vi "AlliGator ucno_objective function phasor calibration.vi"(3 "output control":T1, 4 "data":variant, 5 "X":dbl[](array[numeric])) -> (0 "error out":errorcluster, 1 "gradient":dbl[](array[numeric]), 2 "f(X)":dbl)   [LabVIEW 2021, in "AlliGator Phasor Calibration.lvlib"]
doc: "Minimization function used to search for the optimal calibration based on two references."
uses:
  Variant/Variant to Data/Variant to [DBL].vi
  AlliGator Phasor Calibration.lvlib
  Variant/Variant to Data/Variant to Data.lvlib
panel:
  # "see the AlliGator License on the block diagram (Ctrl+E or Window:Show Block Diagram)"
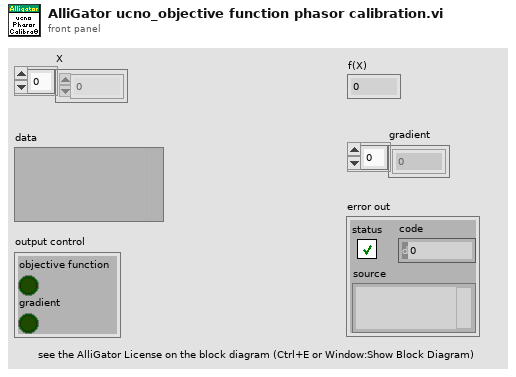
[diagram p1: front panel]
types:
  T1 = cluster{"objective function":bool, "gradient":bool}
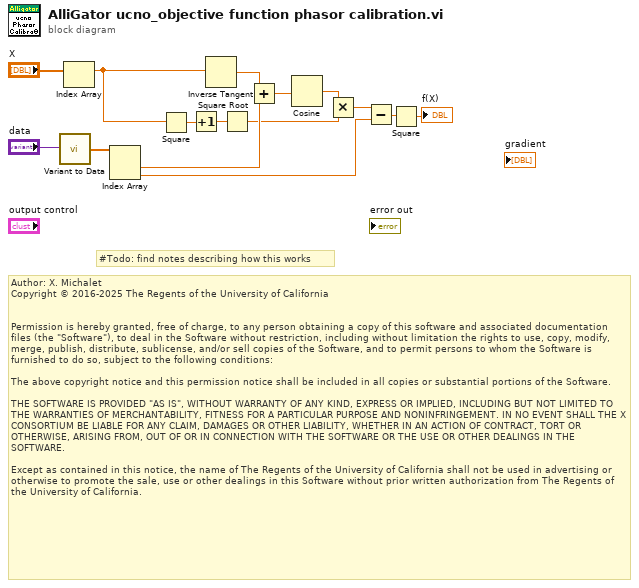
[diagram p0: block diagram]
diagram:
  # "Author: X. Michalet\nCopyright © 2016-2025 The Regents of the University of California\n \n\nPermission is hereby granted, free of charge, to any person obtaining a copy of this software and associated documentation files (the \"Software\"), to deal in the Software without restriction, including without limitation the rights to use, copy, modify, merge, publish, distribute, sublicense, and/or sell copies of the Software, and to permit persons to whom the Software is furnished to do so, subject to the following conditions:\n\nThe above copyright notice and this permission notice shall be included in all copies or substantial portions of the Software.\n\nTHE SOFTWARE IS PROVIDED \"AS IS\", WITHOUT WARRANTY OF ANY KIND, EXPRESS OR IMPLIED, INCLUDING BUT NOT LIMITED TO THE WARRANTIES OF MERCHANTABILITY, FITNESS FOR A PARTICULAR PURPOSE AND NONINFRINGEMENT. IN NO EVENT SHALL THE X CONSORTIUM BE LIABLE FOR ANY CLAIM, DAMAGES OR OTHER LIABILITY, WHETHER IN AN ACTION OF CONTRACT, TORT OR OTHERWISE, ARISING FROM, OUT OF OR IN CONNECTION WITH THE SOFTWARE OR THE USE OR OTHER DEALINGS IN THE SOFTWARE.\n\nExcept as contained in this notice, the name of The Regents of the University of California shall not be used in advertising or otherwise to promote the sale, use or other dealings in this Software without prior written authorization from The Regents of the University of California."
  # "#Todo: find notes describing how this works"
  n1 = call-poly "Variant to Data.vi"("Variant"="data") -> ("Value"=w14:dbl[])  [unwired: 8 in]
  n2 = Index Array(array="X") -> (element=w2:dbl)  [unwired: 1 in]
  n3 = Index Array(array=w14) -> (element #1=w12:dbl, element #2=w4:dbl)  [unwired: 2 in]
  n4 = Square(x=w2) -> (x^2=w9:dbl)
  n5 = Increment(x=w9) -> (x+1=w8:dbl)
  n6 = Inverse Tangent(1:w2) -> (0:w13:dbl)
  n7 = Square Root(x=w8) -> (sqrt(x)=w6:dbl)
  n8 = Add(x=w13, y=w12) -> (x+y=w11:dbl)
  n9 = Cosine(x=w11) -> (cos(x)=w7:dbl)
  n10 = Multiply(x=w7, y=w6) -> (x*y=w5:dbl)
  n11 = Subtract(x=w5, y=w4) -> (x-y=w3:dbl)
  n12 = Square(x=w3) -> (x^2=→"f(X)":dbl)
